vi "Read Device Info.vi"(8 "error in (no error)":errorcluster, 11 "PicoScope 3000a in":refnum<class "PicoScope 3000a.lvclass">) -> (0 "error out":errorcluster, 2 "Device Info":T1, 3 "PicoScope 3000a out":refnum<class "PicoScope 3000a.lvclass">)   [LabVIEW 2018, in "PicoScope 3000a.lvlib" / "PicoScope 3000a.lvclass"]
uses:
  PicoScope 3000a.lvclass
  PicoScope 3000a.lvclass/PicoScope 3000a.ctl
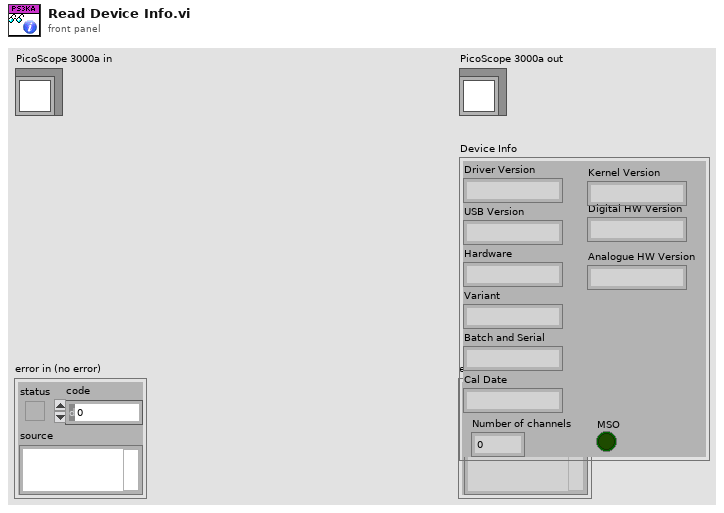
[diagram p1: front panel]
types:
  T1 = cluster{"Driver Version":string, "USB Version":string, "Hardware":string, "Variant":string, "Batch and Serial":string, "Cal Date":string, "Kernel Version":string, "Digital HW Version":string, "Analogue HW Version":string, "MSO":bool, "Number of channels":i16}
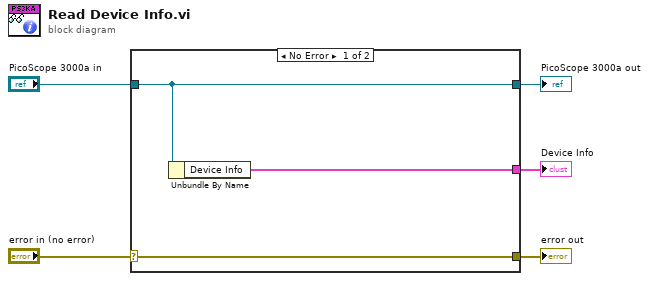
[diagram p0: block diagram]
diagram:
  n1 = case shown="No Error" "error in (no error)" {
    selector: "error in (no error)" -> [w8 w9]
    tunnel: [w8 w9] -> w4
    tunnel: [w7 w10] -> w2
    tunnel: "PicoScope 3000a in" -> [w7 w10]
    tunnel: [w6 _] -> w1
    frame No Error {
      n2 = Unbundle By Name(w7) -> ("Device Info"=w6:T1)
    }
    frame Error {
    }
  }
  "error out" <- w4
  "PicoScope 3000a out" <- w2
  "Device Info" <- w1
